vi "ROS_Master_getSystemStateReply.vi"(3 "ROS_Master in":T1) -> (0 "XML":string)   [LabVIEW 2012]
doc: "Returns XML for the system state reply"
uses:
  <userlib>/ROSforLV/ROS/Code/ROS_Master/ROS_Master.ctl
  <userlib>/ROSforLV/ROS/Code/ROS_Master/ROS_Topic.ctl
  <userlib>/ROSforLV/ROS/Code/ROS_Master/ROS_Node.ctl
  <userlib>/ROSforLV/ROS/Code/ROS_Master/ROS_Service.ctl
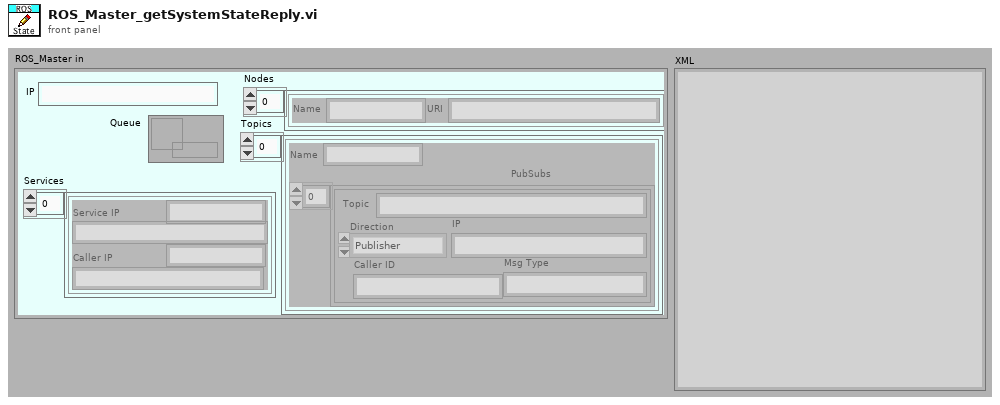
[diagram p1: front panel]
types:
  T1 = typedef "ROS_Master.ctl" = cluster{"IP":string, "Topics":cluster{"Name":string, "PubSubs":T2[]}[], "Nodes":T3[], "Services":T4[], "Queue":refnum<queue>}
  T2 = typedef "ROS_Topic.ctl" = cluster{"Caller ID":string, "IP":string, "Msg Type":string, "Direction":enum16{"Publisher", "Subscriber"}, "Topic":string}
  T3 = typedef "ROS_Node.ctl" = cluster{"Name":string, "URI":string}
  T4 = typedef "ROS_Service.ctl" = cluster{"Service":string, "Service IP":string, "Caller IP":string, "Caller ID":string}
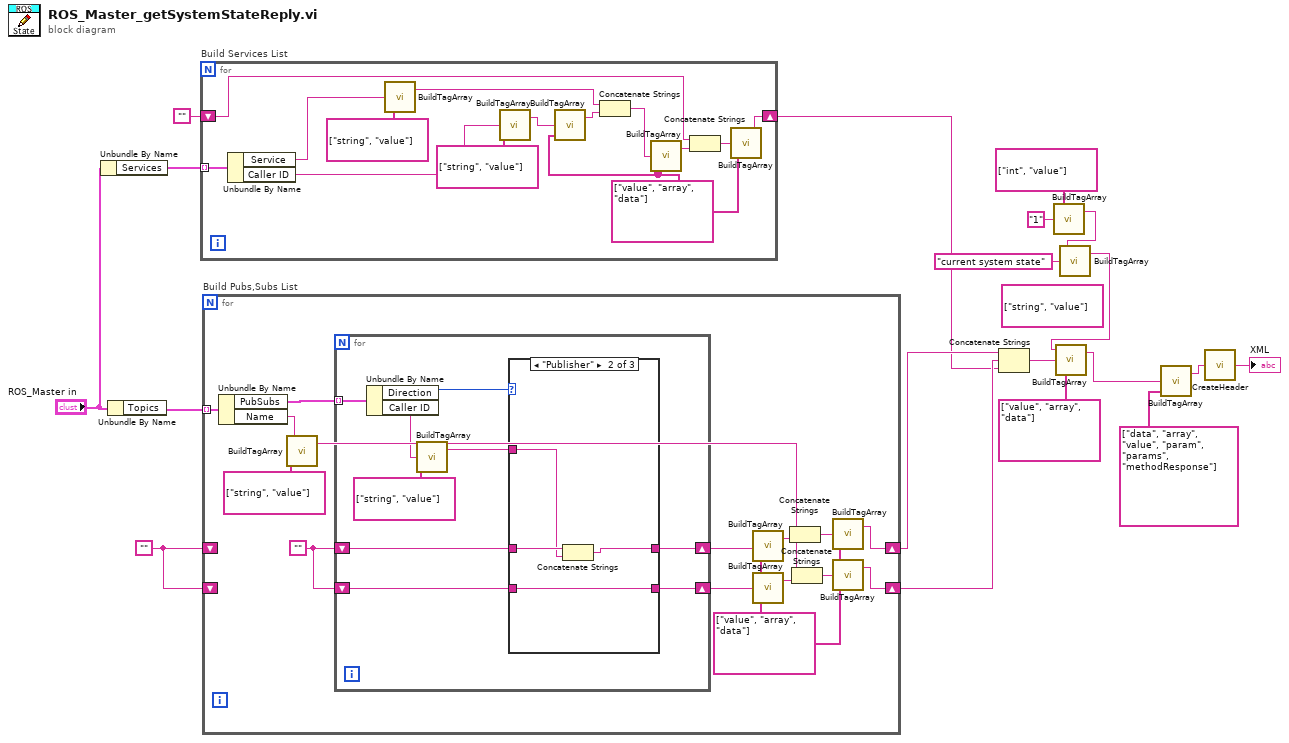
[diagram p0: block diagram]
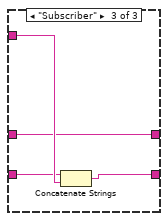
[diagram p3: hidden frame]
diagram:
  (unwired) string[] ["string", "value"] ("tags")
  w18 = ""
  n1 = Unbundle By Name("ROS_Master in") -> ("Services"=w17:T4[])
  n2 = Unbundle By Name("ROS_Master in") -> ("Topics"=w19:cluster{"Name":string, "PubSubs":T2[]}[])
  n3 = for "Build Services List" {
    tunnel: w17 -> [w33] mode=indexing
    shift-right: [w20] -> w13
    shift-left: "" -> [w21]
    w26 = string[] ["value", "array", "data"] ("tags")
    n4 = Unbundle By Name(w33) -> ("Service"=w28:string, "Caller ID"=w27:string)
    n5 = call <userlib>:"BuildTagArray.vi"("tags"=string[] ["string", "value"], "value"=w28) -> ("string out"=w23:string)  [unwired: 2 in]
    n6 = call <userlib>:"BuildTagArray.vi"("tags"=string[] ["string", "value"], "value"=w27) -> ("string out"=w25:string)  [unwired: 2 in]
    n7 = call <userlib>:"BuildTagArray.vi"("tags"=w26, "value"=w25) -> ("string out"=w24:string)  [unwired: 2 in]
    n8 = Concatenate Strings(w23, w24) -> (w22:string)
    n9 = call <userlib>:"BuildTagArray.vi"("tags"=w26, "value"=w22) -> ("string out"=w31:string)  [unwired: 2 in]
    n10 = Concatenate Strings(w21, w31) -> (w30:string)
    n11 = call <userlib>:"BuildTagArray.vi"("tags"=w26, "value"=w30) -> ("string out"=w20:string)  [unwired: 2 in]
  }
  n12 = for "Build Pubs,Subs List" {
    tunnel: w19 -> [w48] mode=indexing
    shift-right: [w34] -> w15
    shift-left: w18 -> [_]
    shift-right: [w35] -> w14
    shift-left: w18 -> [_]
    w36 = string[] ["value", "array", "data"] ("tags")
    w44 = ""
    n13 = Unbundle By Name(w48) -> ("PubSubs"=w47:T2[], "Name"=w46:string)
    n14 = call <userlib>:"BuildTagArray.vi"("tags"=string[] ["string", "value"], "value"=w46) -> ("string out"=w38:string)  [unwired: 2 in]
    n15 = for {
      tunnel: w47 -> [w57] mode=indexing
      shift-right: [w50] -> w43
      shift-left: w44 -> [w52]
      shift-right: [w49] -> w42
      shift-left: w44 -> [w51]
      n16 = Unbundle By Name(w57) -> ("Direction"=w56:enum16{"Publisher", "Subscriber"}, "Caller ID"=w54:string)
      n17 = call <userlib>:"BuildTagArray.vi"("tags"=string[] ["string", "value"], "value"=w54) -> ("string out"=w53:string)  [unwired: 2 in]
      n18 = case shown="\"Publisher\"" w56 {
        tunnel: w53 -> [_ w62 w67]
        tunnel: w52 -> [w59 w63 w64]
        tunnel: w51 -> [w58 w60 w66]
        tunnel: [w59 w61 w64] -> w50
        tunnel: [w58 w60 w65] -> w49
        frame Default {
        }
        frame "Publisher" {
          n19 = Concatenate Strings(w63, w62) -> (w61:string)
        }
        frame "Subscriber" {
          n20 = Concatenate Strings(w66, w67) -> (w65:string)
        }
      }
    }
    n21 = call <userlib>:"BuildTagArray.vi"("tags"=w36, "value"=w43) -> ("string out"=w41:string)  [unwired: 2 in]
    n22 = call <userlib>:"BuildTagArray.vi"("tags"=w36, "value"=w42) -> ("string out"=w39:string)  [unwired: 2 in]
    n23 = Concatenate Strings(w38, w41) -> (w40:string)
    n24 = Concatenate Strings(w38, w39) -> (w37:string)
    n25 = call <userlib>:"BuildTagArray.vi"("tags"=w36, "value"=w40) -> ("string out"=w34:string)  [unwired: 2 in]
    n26 = call <userlib>:"BuildTagArray.vi"("tags"=w36, "value"=w37) -> ("string out"=w35:string)  [unwired: 2 in]
  }
  n27 = Concatenate Strings(w15, w14, w13) -> (w12:string)
  n28 = call <userlib>:"BuildTagArray.vi"("tags"=string[] ["int", "value"], "value"="1") -> ("string out"=w10:string)  [unwired: 2 in]
  n29 = call <userlib>:"BuildTagArray.vi"("value"="current system state", "string in"=w10) -> ("string out"=w6:string)  [unwired: 2 in]
  n30 = call <userlib>:"BuildTagArray.vi"("tags"=string[] ["value", "array", "data"], "value"=w12, "string in"=w6) -> ("string out"=w2:string)  [unwired: 1 in]
  n31 = call <userlib>:"BuildTagArray.vi"("tags"=string[] ["data", "array", "value", "param", "params", "methodResponse"], "value"=w2) -> ("string out"=w4:string)  [unwired: 2 in]
  n32 = call <userlib>:"CreateHeader.vi"("Content"=w4) -> ("XML"=→"XML":string)
